vi "Ref_2_ch_11-20.vi"(0 "Control  Ch 13":refnum<vi>, 1 "Control  Ch 14":refnum<vi>, 2 "Control  Ch 15":refnum<vi>, 3 "Init_F":bool=TRUE, 4 "Control  Ch 16":refnum<vi>, 5 "Control  Ch 17":refnum<vi>, 6 "Control  Ch 18":refnum<vi>, 7 "error in":errorcluster, 8 "Control  Ch 12":refnum<vi>, 9 "Control  Ch 20":refnum<vi>, 10 "Control  Ch 11":refnum<vi>, 12 "Control  Ch 19":refnum<vi>) -> (16 "Control  Ch 20 out":refnum<vi>, 17 "Control  Ch 11 out":refnum<vi>, 18 "Control  Ch 19 out":refnum<vi>, 19 "Control  Ch 12 out":refnum<vi>, 21 "Control  Ch 18 out":refnum<vi>, 22 "Control  Ch 17 out":refnum<vi>, 23 "Control  Ch 16 out":refnum<vi>, 24 "Control  Ch 15 out":refnum<vi>, 25 "Control  Ch 14 out":refnum<vi>, 26 "Control  Ch 13 out":refnum<vi>, 27 "error out":errorcluster)   [LabVIEW 2017]
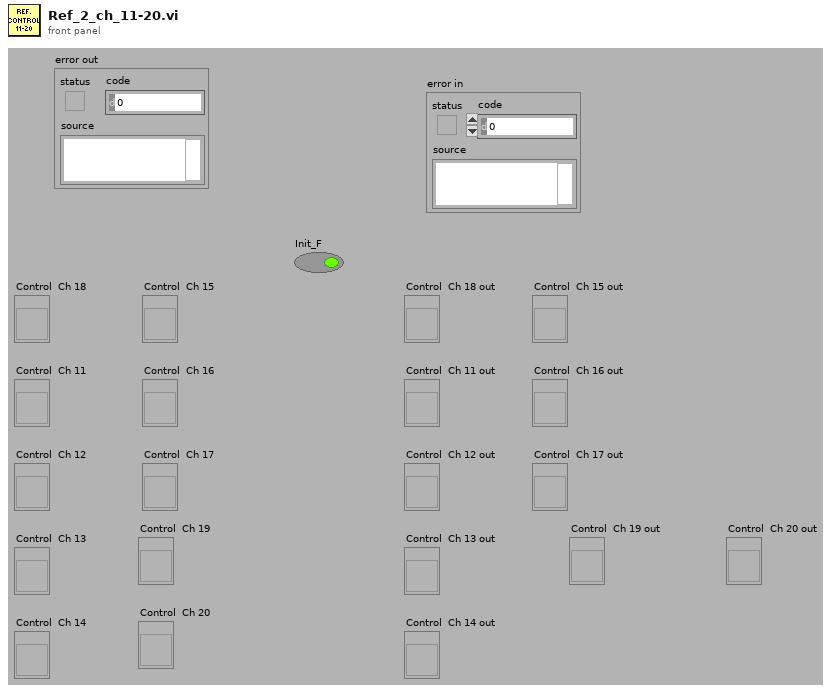
[diagram p1: front panel]
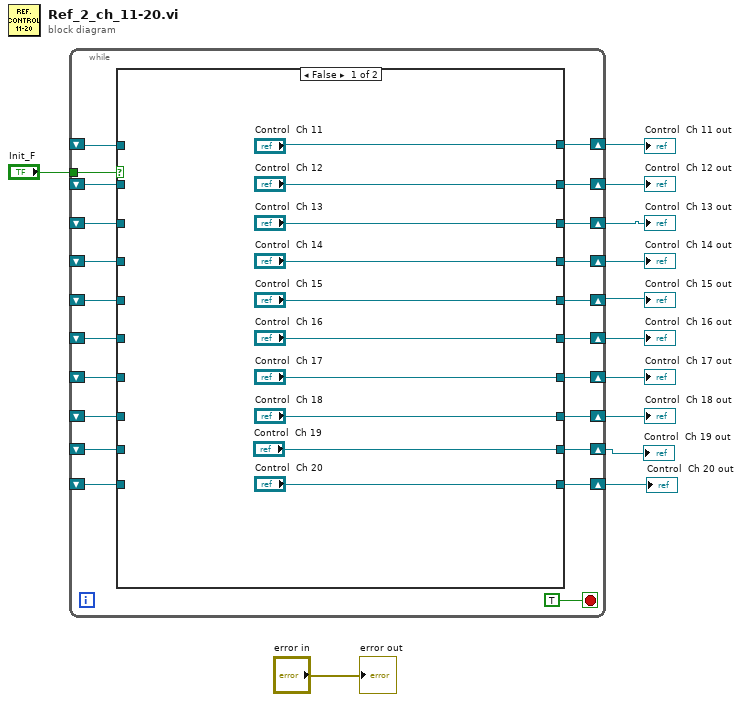
[diagram p0: block diagram]
diagram:
  n1 = while {
    shift-right: [w33] -> w10
    shift-left: _ -> [w32]
    tunnel: "Init_F" -> [w31]
    shift-right: [w30] -> w9
    shift-left: _ -> [w23]
    shift-right: [w29] -> w6
    shift-left: _ -> [w22]
    shift-right: [w28] -> w8
    shift-left: _ -> [w17]
    shift-right: [w27] -> w7
    shift-left: _ -> [w21]
    shift-right: [w26] -> w5
    shift-left: _ -> [w20]
    shift-right: [w25] -> w4
    shift-left: _ -> [w19]
    shift-right: [w24] -> w3
    shift-left: _ -> [w18]
    shift-right: [w16] -> w2
    shift-left: _ -> [w14]
    shift-right: [w15] -> w1
    shift-left: _ -> [w13]
    stop <- TRUE stop-if-true
    n2 = case shown="False" w31 {
      tunnel: ["Control  Ch 11" w54] -> w33
      tunnel: w32 -> [_ w54]
      tunnel: ["Control  Ch 12" w47] -> w30
      tunnel: ["Control  Ch 13" w48] -> w29
      tunnel: ["Control  Ch 14" w49] -> w28
      tunnel: ["Control  Ch 15" w50] -> w27
      tunnel: ["Control  Ch 16" w51] -> w26
      tunnel: ["Control  Ch 17" w52] -> w25
      tunnel: ["Control  Ch 18" w53] -> w24
      tunnel: w23 -> [_ w47]
      tunnel: w22 -> [_ w48]
      tunnel: w21 -> [_ w50]
      tunnel: w20 -> [_ w51]
      tunnel: w19 -> [_ w52]
      tunnel: w18 -> [_ w53]
      tunnel: w17 -> [_ w49]
      tunnel: ["Control  Ch 19" w46] -> w16
      tunnel: ["Control  Ch 20" w45] -> w15
      tunnel: w14 -> [_ w46]
      tunnel: w13 -> [_ w45]
      frame False {
      }
      frame True {
      }
    }
  }
  "Control  Ch 18 out" <- w3
  "Control  Ch 17 out" <- w4
  "Control  Ch 16 out" <- w5
  "Control  Ch 15 out" <- w7
  "Control  Ch 14 out" <- w8
  "Control  Ch 13 out" <- w6
  "Control  Ch 12 out" <- w9
  "Control  Ch 11 out" <- w10
  "Control  Ch 19 out" <- w2
  "Control  Ch 20 out" <- w1
  "error out" <- "error in"
